vi "Dlg Save File.vi"(8 "error in":errorcluster, 11 "JSON in":refnum<class "JSON.lvclass">) -> (0 "error out":errorcluster, 2 "cancelled":bool, 3 "JSON out":refnum<class "JSON.lvclass">)   [LabVIEW 2017, in "Report_lib.lvlib" / "JSON.lvclass"]
doc: "This Dynamic method for call\nSave Dialog window"
uses:
  JSON.lvclass
  JSON.lvclass/JSON.ctl
panel:
  out "selected path":path
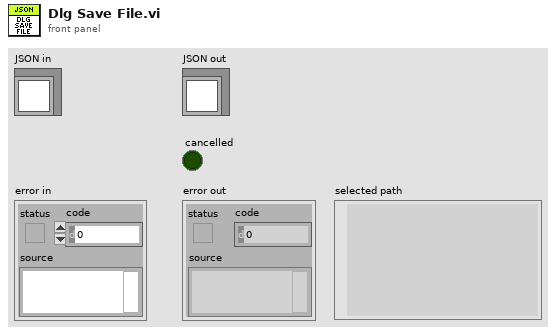
[diagram p1: front panel]
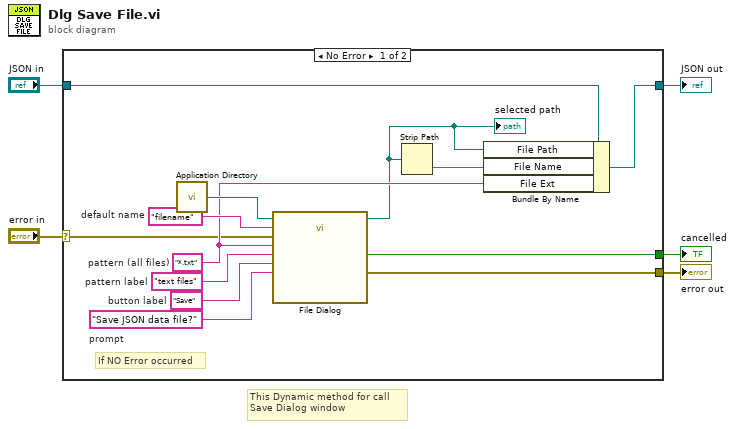
[diagram p0: block diagram]
diagram:
  # "This Dynamic method for call\nSave Dialog window"
  n1 = case shown="No Error" "error in" {
    selector: "error in" -> [w8 w20]
    tunnel: [w7 w20] -> w4
    tunnel: [w9 w19] -> w2
    tunnel: "JSON in" -> [w10 w19]
    tunnel: [w6 _] -> w1
    frame No Error {
      w14 = "text files"  # pattern label
      w15 = "Save JSON data file?"  # prompt
      w16 = "Save"  # button label
      w12 = "*.txt"  # pattern (all files)
      w17 = "filename"  # default name
      # "If NO Error occurred"
      n2 = call <vilib>:"Application Directory.vi"() -> ("Application Directory"=w18:path)
      n3 = call "File Dialog"("start path"=w18, "prompt"=w15, "button label"=w16, "default name"=w17, "error in"=w8, "pattern (all files)"=w12, "pattern label"=w14) -> ("selected path"=w11:path, "cancelled"=w6:bool, "error out"=w7:errorcluster)  [unwired: 5 in, 1 out]
      "selected path" <- w11
      n4 = Strip Path(path=w11) -> (name=w13:string)  [unwired: 1 out]
      n5 = Bundle By Name(cluster=w10, "File Path"=w11, "File Name"=w13, "File Ext"=w12) -> (w9:refnum<class "JSON.lvclass">)
    }
    frame Error {
    }
  }
  "error out" <- w4
  "JSON out" <- w2
  "cancelled" <- w1
